vi "SECoP_dataGetStructName.vi"(7 "Position":u32, 8 "error in (no error)":errorcluster, 10 "SECoP_dataPtr in":T1 {"ptr64" format="%.0x"; "ptr32" format="%.0x"}, 11 "DLL path (in)":T2) -> (0 "error out":errorcluster, 1 "struct_name":string, 3 "DLL path (out)":T2)   [LabVIEW 2023, in "SECoP.lvlib"]
doc: "Call <b>\"SECoP_dataGetStructName.vi\"</b> to access the item names of a structured data type.\n\n<b>DLL path</b> input and output of cluster from \"SECoP-Initialize.vi\"\n<b>SECoP_dataPtr</b> data to access\n<b>Position</b> points to a virtual flattened entry of the data type (<b>Position</b> of struct plus zero based index up to <b>\"SECoP_dataGetStructCount.vi\"-1</b>)\n<b>struct_name</b> item name"
uses:
  SECoP.lvlib
  SECoP-libraries.ctl
  SECoP-data.ctl
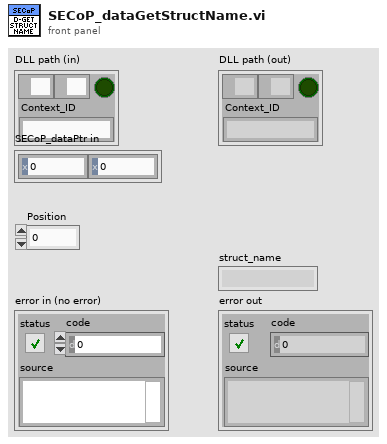
[diagram p1: front panel]
types:
  T1 = typedef "SECoP.lvlib/SECoP-data.ctl" = cluster{"ptr32":u32, "ptr64":u64}
  T2 = typedef "SECoP.lvlib/SECoP-libraries.ctl" = cluster{"serverDLL":path, "variantDLL":path, "cleanup_mode":bool, "Context_ID":string}
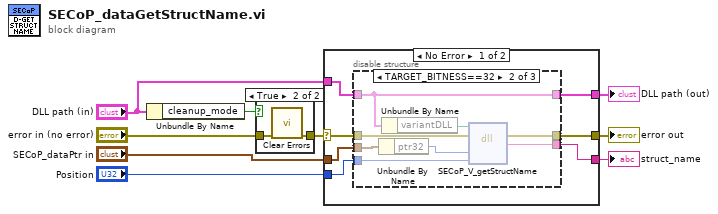
[diagram p0: block diagram]
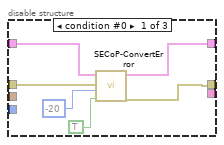
[diagram p3: hidden frame]
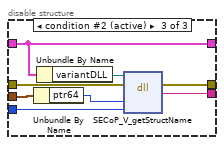
[diagram p4: hidden frame]
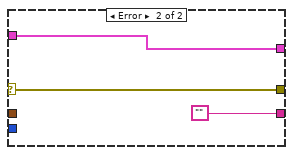
[diagram p5: hidden frame]
diagram:
  n1 = Unbundle By Name("DLL path (in)") -> ("cleanup_mode"=w6:bool)
  n2 = case shown="True" w6 {
    tunnel: "error in (no error)" -> [w10 w12]
    tunnel: [w10 w11] -> w4
    frame False {
    }
    frame True {
      n3 = call <vilib>:"Clear Errors.vi"("error in (no error)"=w12) -> ("error out"=w11:errorcluster)  [unwired: 5 in, 1 out]
    }
  }
  n4 = case shown="No Error" w4 {
    selector: w4 -> [w19 w43]
    tunnel: "DLL path (in)" -> [w18 w44]
    tunnel: [w15 w44] -> w8
    tunnel: [w16 w43] -> w7
    tunnel: "Position" -> [w17 _]
    tunnel: [w14 ""] -> w2
    tunnel: "SECoP_dataPtr in" -> [w13 _]
    frame No Error {
      n5 = disable-structure shown="TARGET_BITNESS==32" {
        disable-tunnel: w19 -> [w24 w33 w41]
        disable-tunnel: w18 -> [w25 w27 w35]
        disable-tunnel: w17 -> [_ w32 w40]
        disable-tunnel: [w23 w31 w39] -> w16
        disable-tunnel: [w20 w27 w35] -> w15
        disable-tunnel: [_ w30 w38] -> w14
        disable-tunnel: w13 -> [_ w29 w37]
        frame condition #0 {
          n6 = call "SECoP-ConvertError.vi"("return is boolean"=TRUE, "return code"=-20, "error in (no error)"=w24, "DLL path (in)"=w25) -> ("error out"=w23:errorcluster, "DLL path (out)"=w20:T2)  [unwired: 6 in]
        }
        frame condition #1 {
          n7 = Unbundle By Name(w29) -> ("ptr32"=w28:u32)
          n8 = Unbundle By Name(w27) -> ("variantDLL"=w26:path)
          n9 = dll-call lib="Z:/Praktische_Aufgaben/SECoP-LabVIEW2015/32bit/SECoP32.dll" fn="SECoP_V_getStructName"(path in=w26, error in=w33, "pData"=w28, "uPosition"=w32) -> (error out=w31:errorcluster, "return type"=w30:string)  [unwired: 3 in, 1 out]
        }
        frame condition #2 (active) {
          n10 = Unbundle By Name(w37) -> ("ptr64"=w36:u64)
          n11 = Unbundle By Name(w35) -> ("variantDLL"=w34:path)
          n12 = dll-call lib="Z:/Praktische_Aufgaben/SECoP-LabVIEW2015/32bit/SECoP32.dll" fn="SECoP_V_getStructName"(path in=w34, error in=w41, "pData"=w36, "uPosition"=w40) -> (error out=w39:errorcluster, "return type"=w38:string)  [unwired: 3 in, 1 out]
        }
      }
    }
    frame Error {
    }
  }
  "DLL path (out)" <- w8
  "error out" <- w7
  "struct_name" <- w2
